vi "Day11-reset_energy_levels.vi"(11 "Energy Levels":i32[][](array[numeric])) -> (3 "Energy Levels out":i32[][](array[numeric]))   [LabVIEW 2021]
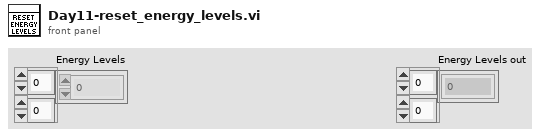
[diagram p1: front panel]
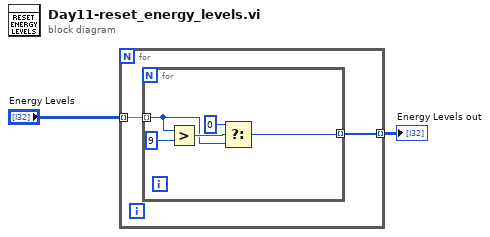
[diagram p0: block diagram]
diagram:
  n1 = for {
    tunnel: "Energy Levels" -> [w4] mode=indexing
    tunnel: [w3] -> w1 mode=indexing
    n2 = for {
      tunnel: w4 -> [w7] mode=indexing
      tunnel: [w5] -> w3 mode=indexing
      n3 = Greater?(x=w7, y=9) -> (0:w8:bool)
      n4 = Select(t=0, s=w8, f=w7) -> (s? t:f=w5:i32)
    }
  }
  "Energy Levels out" <- w1
